vi "Property Tree Symbol Handler_2.vi"(7 "Save Action":T1=enum."Wire Unbundle", 11 "Tree refs":refnum<vi>[](array[refnum])) -> ()   [LabVIEW 2023]
doc: "Synchronize scroll position and value of registered tree controls."
uses:
  controls/action enum.ctl
panel:
  out "Clicked Item Disabled":bool
  out "Double Click":bool
  out "Source":u32(ring) items=["LabVIEW UI"=0, "ActiveX"=1, "User Event"=25]
  in  "Main Tree":string[](tree)
  in  "Write Tree":string[](tree)
  in  "Read Tree":string[](tree)
  in  "Stop":bool
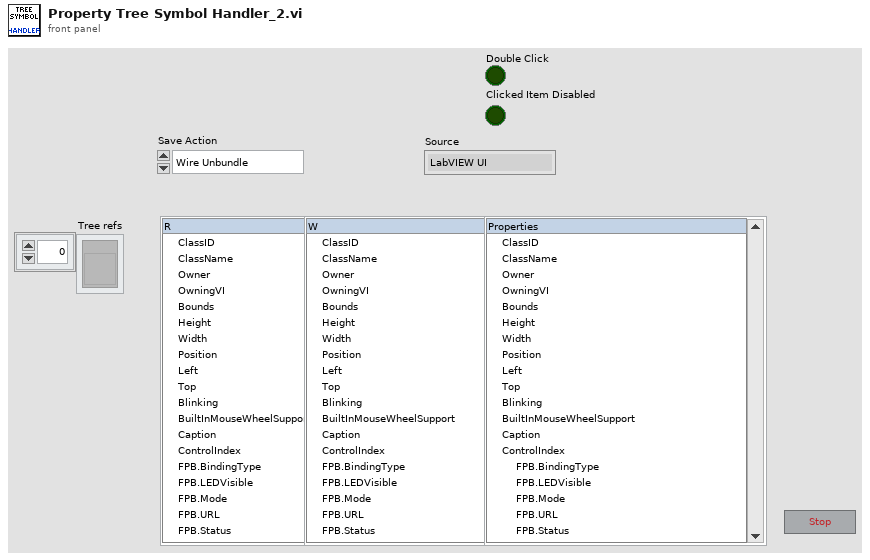
[diagram p1: front panel]
types:
  T1 = typedef "action enum.ctl" = enum16{"[NONE]", "Wire Bundle", "Wire Unbundle", "Terminal Unbundle", "Terminal Bundle", "Bundler Move Up", "Bundler Move Down", "Bundler Insert", "Bundler Remove", "Bundler Remove Unwired", "Bundler Rearrange", "In Place Insert", "In Place Remove", "In Place Remove Unwired", "In Place Rearrange", "Wire Properties", "Wire Method", "Terminal Properties", "Terminal Method", "Property Move Up", "Property Move Down", "Properties Insert", "Properties Remove", "Properties Remove Unwired", "Properties Rearrange", "Method Change", "Class for Constant", "Class For Control", "Class For Node", "Class Name to Clipboard"}
  T2 = enum16{"Init", "Read", "Remove", "Remove or Append", "Append", "Append If New"}
  T3 = cluster{"Tag":string, "Read":bool, "Write":bool, "New":bool}
  T4 = cluster{"Tag":string, "Read":bool, "Write":bool, "New":bool}[]
  T5 = typedef "LVPoint32TypeDef.ctl" = cluster{"Horizontal":i32, "Vertical":i32}
  T6 = typedef "eventsource.ctl" = u32
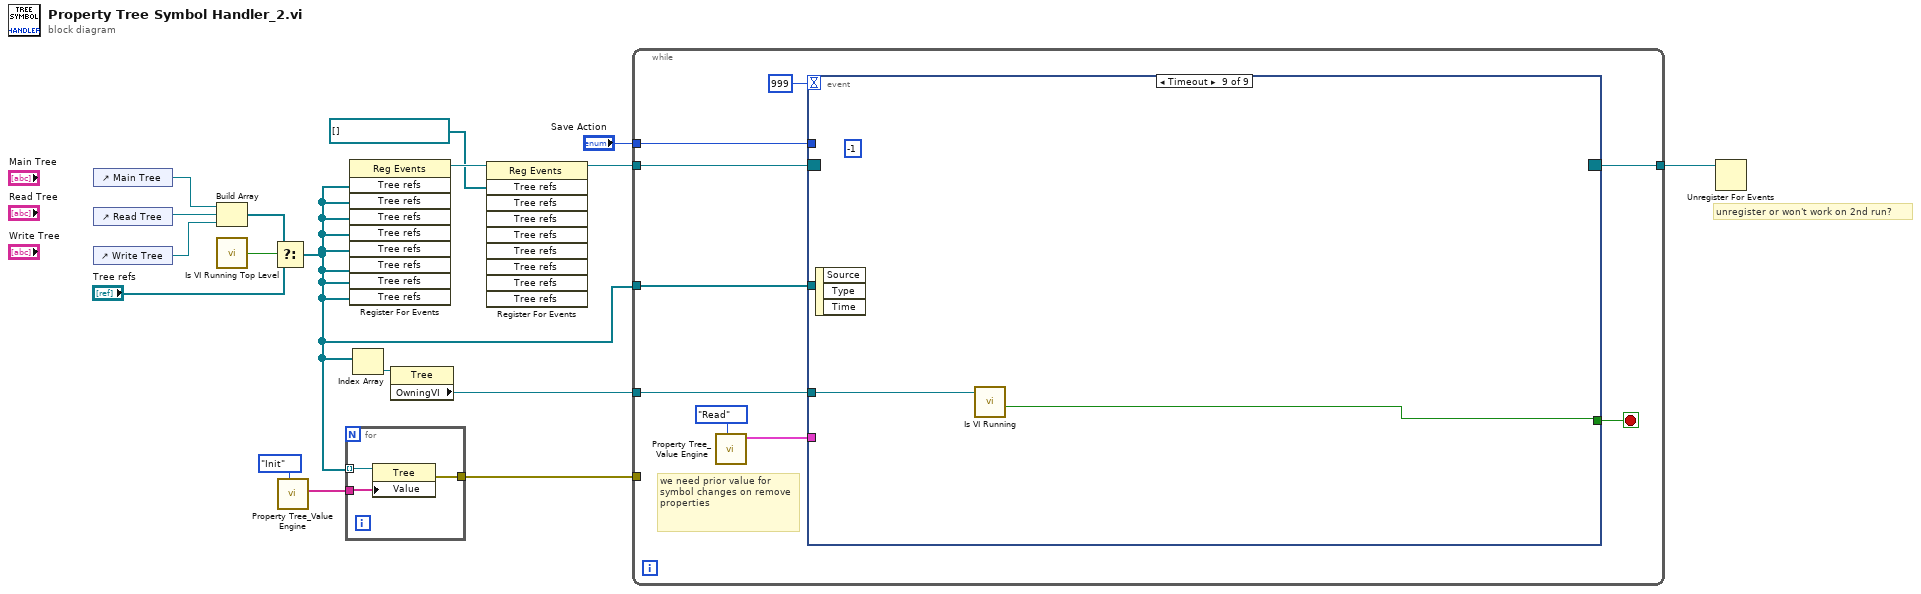
[diagram p0: block diagram]
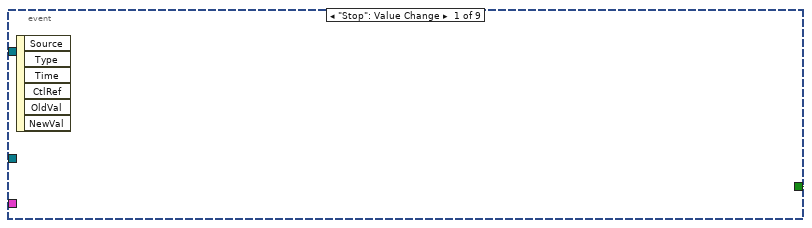
[diagram p2: hidden frame]
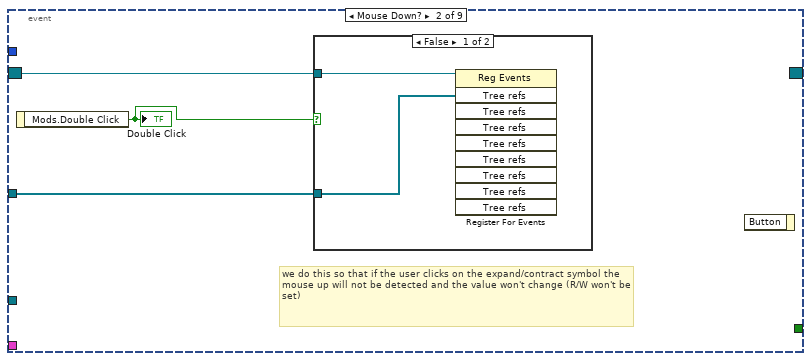
[diagram p3: hidden frame]
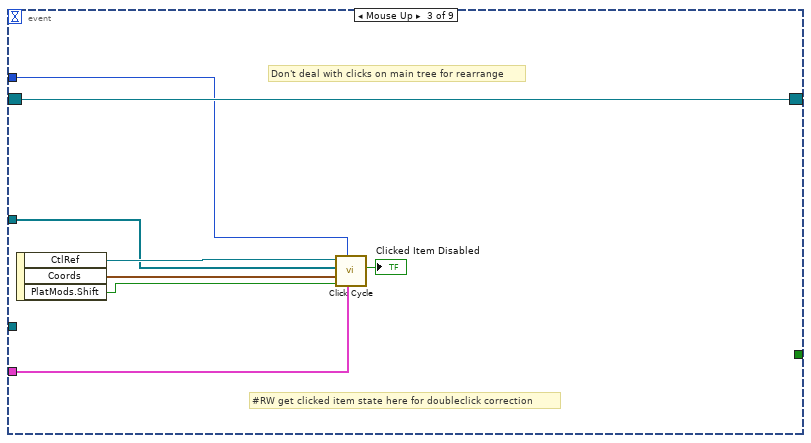
[diagram p5: hidden frame]
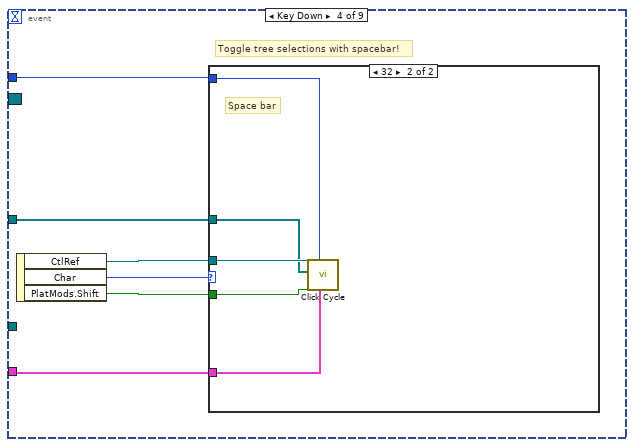
[diagram p6: hidden frame]
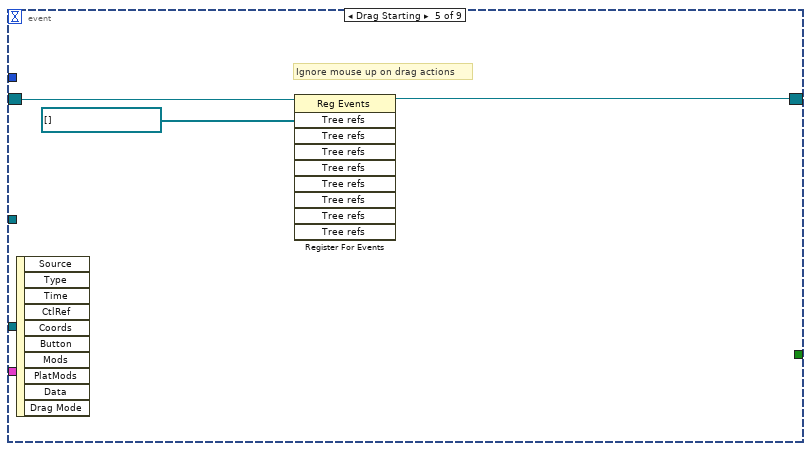
[diagram p8: hidden frame]
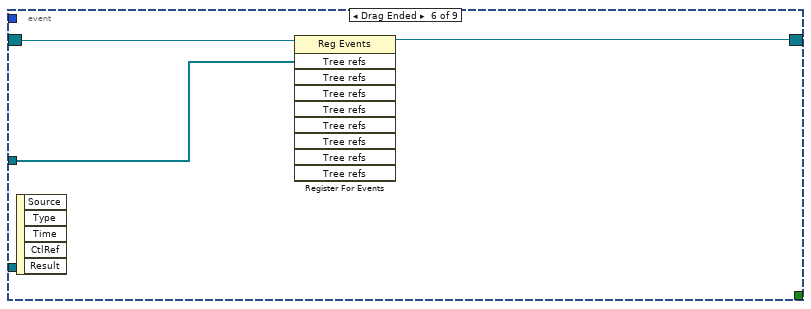
[diagram p9: hidden frame]
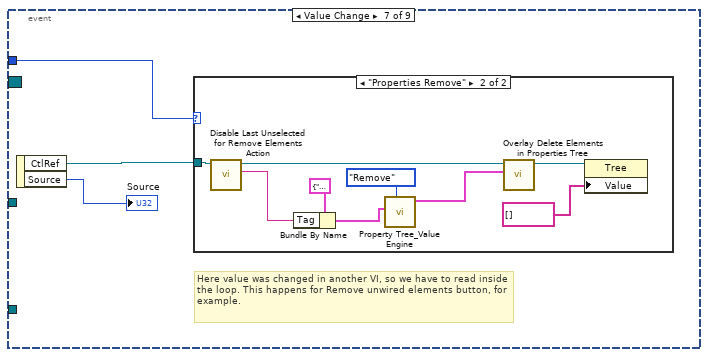
[diagram p10: hidden frame]
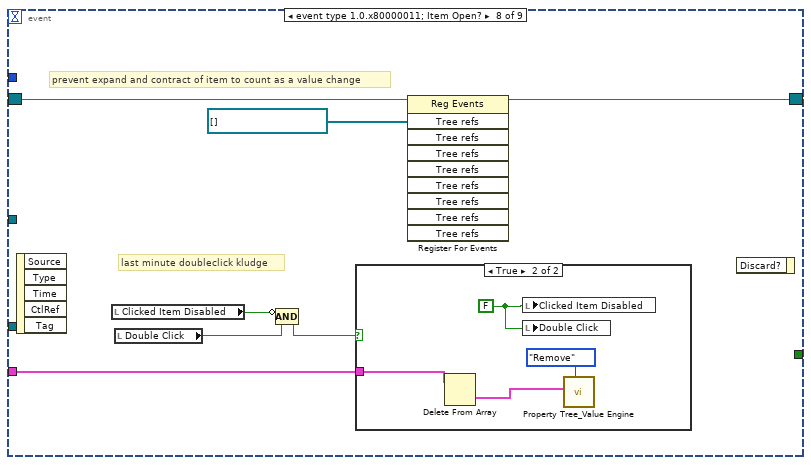
[diagram p12: hidden frame]
diagram:
  # "unregister or won't work on 2nd run?"
  n1 = control-ref of="Main Tree"() -> (w2:refnum<vi>)
  n2 = control-ref of="Read Tree"() -> (w17:refnum<vi>)
  n3 = control-ref of="Write Tree"() -> (w16:refnum<vi>)
  n4 = Build Array(w2, w17, w16) -> (w15:refnum<vi>[])
  n5 = call "Is VI Running Top Level.vi"() -> ("Top Level?"=w7:bool)  [unwired: 5 in]
  n6 = Select(t=w15, s=w7, f="Tree refs") -> (s? t:f=w1:refnum<vi>[])
  n7 = call "Property Tree_Value Engine.vi"("Save Action"=T2."Init" ("Action")) -> ("Tag Array"=w10:string[])  [unwired: 8 in, 2 out]
  n8 = for {
    tunnel: w10 -> [w19]
    tunnel: w1 -> [w20] mode=indexing
    tunnel: [w18] -> w9
    n9 = property class="Tree"(reference=w20, "Value"=w19) -> (error out=w18:errorcluster)  [unwired: 1 in, 1 out]
  }
  n10 = register-events(w1, w1, w1, w1, w1, w1, w1, w1) -> (reference out=w5:refnum<event-registration>)  [unwired: 2 in, 1 out]
  n11 = Index Array(array=w1) -> (element=w13:refnum<vi>)  [unwired: 1 in]
  n12 = property class="Tree"(reference=w13) -> ("OwningVI"=w12:refnum<vi>)  [unwired: 1 in, 2 out]
  n13 = register-events(reference=w5, refnum<vi>[] [] ("event source")) -> (reference out=w4:refnum<event-registration>)  [unwired: 8 in, 1 out]
  n14 = while {
    tunnel: w4 -> [w28]
    tunnel: w12 -> [w27]
    tunnel: w1 -> [w26]
    tunnel: w9 -> [_]
    tunnel: "Save Action" -> [w25]
    tunnel: [w24] -> w6
    stop <- w29 stop-if-true
    # "we need prior value for symbol changes on remove properties"
    n15 = call "Property Tree_Value Engine.vi"("Save Action"=T2."Read" ("Action")) -> ("Property Array Out"=w22:T4)  [unwired: 8 in, 2 out]
    n16 = event shown="[8] Timeout" {
      selector: w28 -> [_ w33 w43 _ w57 w60 _ w79 _]
      dyn-events: [_ _ w43 _ w56 w59 _ w78 _] -> w24
      timeout: 999 -> [_ _ _ _ _ _ _ _ _]
      tunnel: ["Stop" _ _ _ _ _ _ _ w84] -> w29
      tunnel: w27 -> [_ _ _ _ _ _ _ _ w85]
      tunnel: w26 -> [_ w32 w40 w47 _ w58 _ _ _]
      tunnel: w25 -> [_ _ w38 w46 _ _ w62 _ _]
      tunnel: w22 -> [_ _ w39 w44 _ _ _ w76 _]
      event "Stop": Value Change {
        n17 = event-data() -> ()  [unwired: 1 in, 6 out]
      }
      event Mouse Down? {
        # "we do this so that if the user clicks on the expand/contract symbol the mouse up will not be detected and the value won't change (R/W won't be set)"
        n18 = event-data() -> ("Mods.Double Click"=w31:bool)  [unwired: 1 in]
        "Double Click" <- w31
        n19 = case shown="False" w31 {
          tunnel: w33 -> [w35 _]
          tunnel: w32 -> [w34 _]
          frame False {
            n20 = register-events(reference=w35, w34) -> ()  [unwired: 8 in, 2 out]
          }
          frame True {
          }
        }
        n21 = event-data() -> ()  [unwired: 2 in, 1 out]
      }
      event Mouse Up {
        # "#RW get clicked item state here for doubleclick correction"
        # "Don't deal with clicks on main tree for rearrange"
        n22 = event-data() -> ("CtlRef"=w42:refnum<vi>, "Coords"=w37:T5, "PlatMods.Shift"=w41:bool)  [unwired: 1 in]
        n23 = call "Click Cycle.vi"("Prior Property Selection"=w39, "Action"=w38, "Shift"=w41, "Coords"=w37, "All Tree Refs"=w40, "Tree Control Ref"=w42) -> ("Clicked disabled item?"=→"Clicked Item Disabled":bool)  [unwired: 4 in, 1 out]
      }
      event Key Down {
        # "Toggle tree selections with spacebar!"
        n24 = event-data() -> ("CtlRef"=w48:refnum<vi>, "Char"=w49:i16, "PlatMods.Shift"=w45:bool)  [unwired: 1 in]
        n25 = case shown="32" w49 {
          tunnel: w48 -> [_ w54]
          tunnel: w47 -> [_ w53]
          tunnel: w46 -> [_ w52]
          tunnel: w45 -> [_ w51]
          tunnel: w44 -> [_ w50]
          frame 0, Default {
          }
          frame 32 {
            # "Space bar"
            n26 = call "Click Cycle.vi"("Prior Property Selection"=w50, "Action"=w52, "Shift"=w51, "All Tree Refs"=w53, "Tree Control Ref"=w54) -> ()  [unwired: 5 in, 2 out]
          }
        }
      }
      event Drag Starting {
        # "Ignore mouse up on drag actions"
        n27 = event-data() -> ()  [unwired: 1 in, 10 out]
        n28 = register-events(reference=w57, refnum<vi>[] [] ("event source")) -> (reference out=w56:refnum<event-registration>)  [unwired: 8 in, 1 out]
      }
      event Drag Ended {
        n29 = event-data() -> ()  [unwired: 1 in, 5 out]
        n30 = register-events(reference=w60, w58) -> (reference out=w59:refnum<event-registration>)  [unwired: 8 in, 1 out]
      }
      event Value Change {
        # "Here value was changed in another VI, so we have to read inside the loop. This happens for Remove unwired elements button, for example."
        n31 = event-data() -> ("CtlRef"=w61:refnum<vi>, "Source"=→"Source":T6)  [unwired: 1 in]
        n32 = case shown="\"Properties Remove\"" w62 {
          tunnel: w61 -> [_ w71]
          frame Default {
          }
          frame "Properties Remove" {
            n33 = call "Disable Last Unselected for Remove Elements Action.vi"("Tree Ref"=w71) -> ("Removed Item Tag"=w64:string, "Tree Ref Out"=w72:refnum<vi>)  [unwired: 8 in, 1 out]
            n34 = Bundle By Name(cluster=T3 {"Tag"="", "Read"=FALSE, "Write"=FALSE, "New"=FALSE} ("Element"), "Tag"=w64) -> (w66:T3)
            n35 = call "Property Tree_Value Engine.vi"("Save Action"=T2."Remove" ("Action"), "Element"=w66) -> ("Property Array Out"=w67:T4)  [unwired: 7 in, 2 out]
            n36 = call "Overlay Delete Elements in Properties Tree.vi"("Prior Property Array"=w67, "Tree Ref"=w72) -> ("Tree Ref Out"=w70:refnum<vi>)  [unwired: 8 in, 1 out]
            n37 = property class="Tree"(reference=w70, "Value"=string[] []) -> ()  [unwired: 1 in, 2 out]
          }
        }
      }
      event event type 1.0.x80000011; Item Open? {
        # "last minute doubleclick kludge"
        # "prevent expand and contract of item to count as a value change"
        n38 = event-data() -> ()  [unwired: 1 in, 5 out]
        n39 = local read "Clicked Item Disabled"() -> (w75:bool)
        n40 = local read "Double Click"() -> (w74:bool)
        n41 = Compound Arithmetic op=AND(invert w75, w74) -> (w73:bool)
        n42 = case shown="True" w73 {
          tunnel: w76 -> [_ w81]
          frame False {
          }
          frame True {
            w80 = FALSE
            n43 = Delete From Array(array=w81) -> (deleted portion=w82:T3)  [unwired: 2 in, 1 out]
            n44 = local write "Clicked Item Disabled"(w80) -> ()
            n45 = local write "Double Click"(w80) -> ()
            n46 = call "Property Tree_Value Engine.vi"("Save Action"=T2."Remove" ("Action"), "Element"=w82) -> ()  [unwired: 7 in, 3 out]
          }
        }
        n47 = register-events(reference=w79, refnum<vi>[] [] ("event source")) -> (reference out=w78:refnum<event-registration>)  [unwired: 8 in, 1 out]
        n48 = event-data() -> ()  [unwired: 2 in, 1 out]
      }
      event Timeout {
        (unwired) -1
        n49 = event-data() -> ()  [unwired: 1 in, 3 out]
        n50 = call "Is VI Running.vi"("VI in"=w85) -> ("VI Not Running"=w84:bool)  [unwired: 7 in, 3 out]
      }
    }
  }
  n51 = Unregister For Events(event registration refnum=w6) -> ()  [unwired: 1 in, 1 out]
